vi "layout.vi"(0 "reference":refnum<class "PackageNode.lvclass">, 1 "graph":refnum<class "Graph.lvclass">, 2 "graphics":refnum<class "Graphics.lvclass">, 3 "grid":refnum<class "Grid.lvclass">, 5 "error in (no error)":errorcluster) -> (14 "reference out":refnum<class "PackageNode.lvclass">, 19 "error out":errorcluster)   [LabVIEW 2020, in "PackageNode.lvclass"]
doc: "public void draw(Graphics2D g2)"
uses:
  <resource>/Framework/Providers/Open_GDS/UML/PackageNode_class/PackageNode.lvclass
  C:/Program Files (x86)/National Instruments/LabVIEW 2020/resource/Framework/Providers/Open_GDS/UML/RectangularNode_class/RectangularNode.lvclass
  C:/Program Files (x86)/National Instruments/LabVIEW 2020/resource/Framework/Providers/Open_GDS/UML/AbstractNode_class/AbstractNode.lvclass
  <resource>/Framework/Providers/Open_GDS/UML/Grid_class/Grid.lvclass
  <resource>/Framework/Providers/Open_GDS/UML/Graphics_class/Graphics.lvclass
  <resource>/Framework/Providers/Open_GDS/UML/Graph_class/Graph.lvclass
  <resource>/Framework/Providers/Open_GDS/UML/General/Rectangle/Rectangle Rectangle2D.ctl
  <resource>/Framework/Providers/Open_GDS/UML/MultiLineString_class/MultiLineString.lvclass
  <resource>/Framework/Providers/Open_GDS/UML/AbstractNode_class/AbstractNode.lvclass
  <resource>/Framework/Providers/Open_GDS/UML/RectangularNode_class/RectangularNode.lvclass
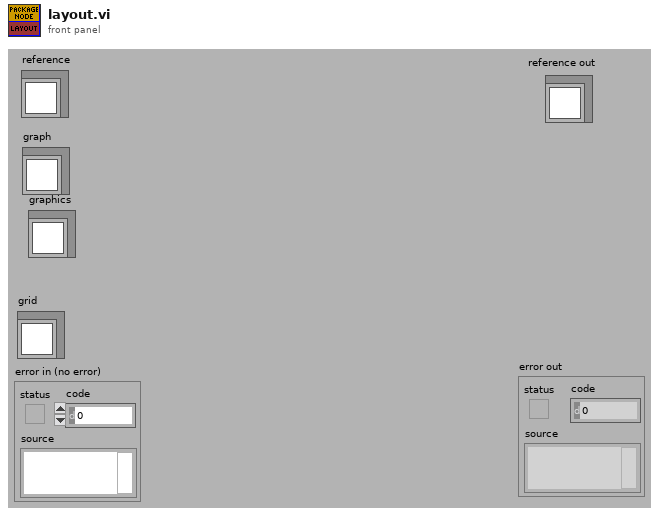
[diagram p1: front panel]
types:
  T1 = typedef "Rectangle Rectangle2D.ctl" = cluster{"x":dbl, "y":dbl, "width":dbl, "height":dbl}
  T2 = typedef "PackageNode.lvclass/ObjectAttributes.ctl" = cluster{"name":string, "contents":refnum<class "MultiLineString.lvclass">, "DEFAULT_TOP_WIDTH":i32, "DEFAULT_TOP_HEIGHT":i32, "DEFAULT_WIDTH":i32, "DEFAULT_HEIGHT":i32, "NAME_GAP":i32, "XGAP":i32, "YGAP":i32, "Collapsed":bool, "Note color":u32, "Justification":u16}
  T3 = typedef "RectangularNode.lvclass/ObjectAttributes.ctl" = cluster{"bounds":T1}
  T4 = typedef "AbstractNode.lvclass/ObjectAttributes.ctl" = cluster{"parent":refnum<class "AbstractNode.lvclass">, "children":refnum<class "AbstractNode.lvclass">[], "Hidden":bool}
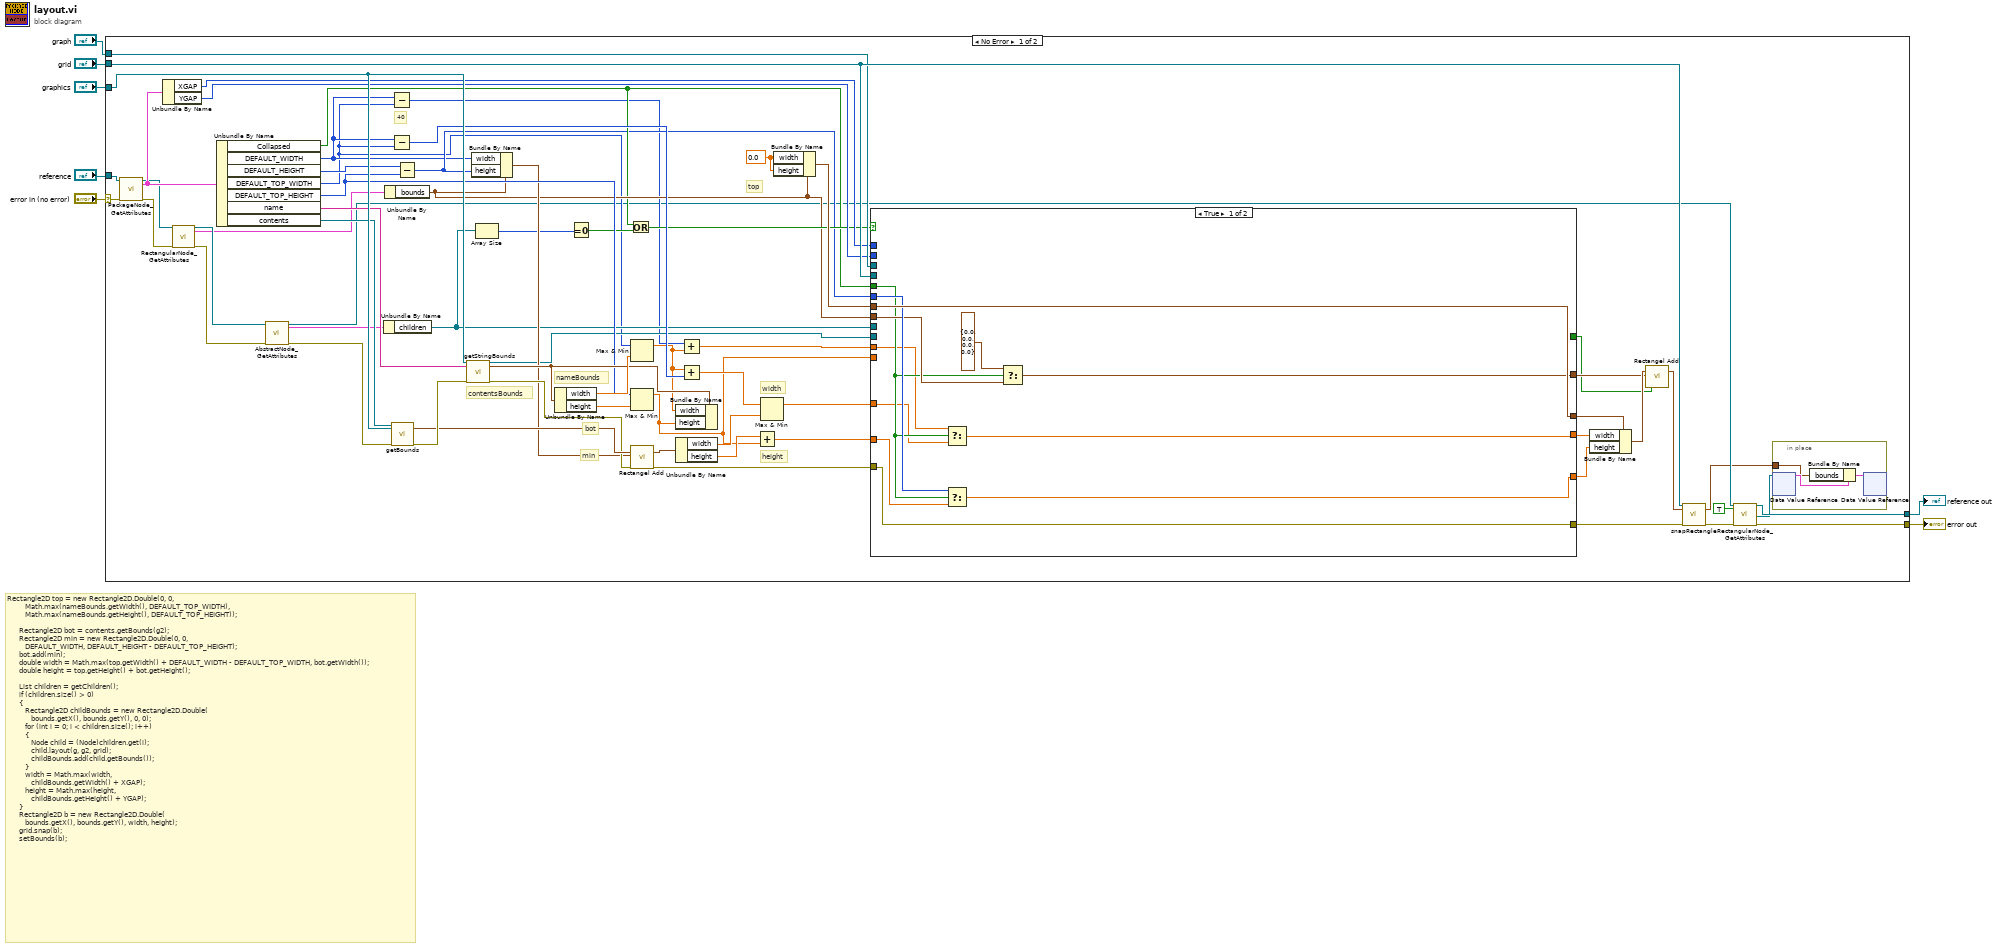
[diagram p0: block diagram]
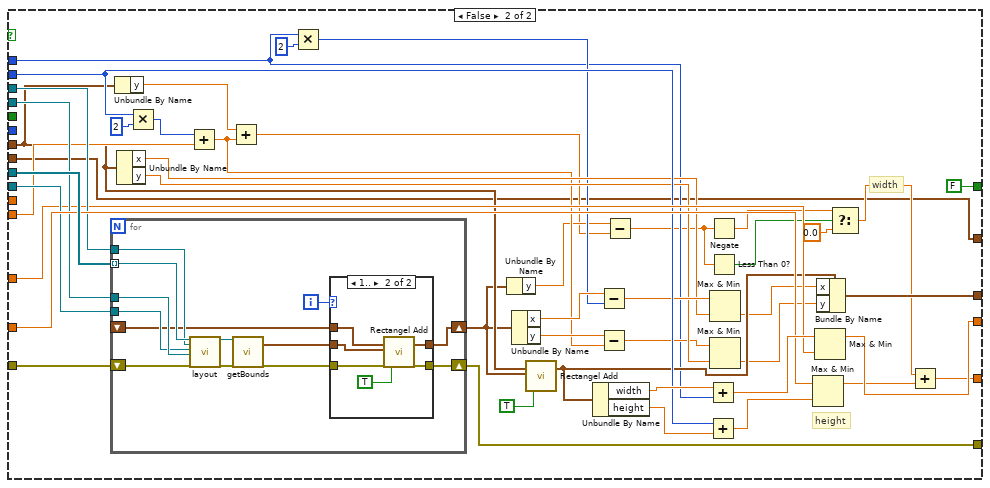
[diagram p2: hidden frame]
diagram:
  # "Rectangle2D top = new Rectangle2D.Double(0, 0,\n         Math.max(nameBounds.getWidth(), DEFAULT_TOP_WIDTH), \n         Math.max(nameBounds.getHeight(), DEFAULT_TOP_HEIGHT));\n\n      Rectangle2D bot = contents.getBounds(g2);\n      Rectangle2D min = new Rectangle2D.Double(0, 0,\n         DEFAULT_WIDTH, DEFAULT_HEIGHT - DEFAULT_TOP_HEIGHT);\n      bot.add(min);\n      double width = Math.max(top.getWidth() + DEFAULT_WIDTH - DEFAULT_TOP_WIDTH, bot.getWidth());\n      double height = top.getHeight() + bot.getHeight();\n\n      List children = getChildren();\n      if (children.size() > 0)\n      {\n         Rectangle2D childBounds = new Rectangle2D.Double(\n            bounds.getX(), bounds.getY(), 0, 0);\n         for (int i = 0; i < children.size(); i++)\n         {\n            Node child = (Node)children.get(i);\n            child.layout(g, g2, grid);\n            childBounds.add(child.getBounds());\n         }\n         width = Math.max(width, \n            childBounds.getWidth() + XGAP);\n         height = Math.max(height, \n            childBounds.getHeight() + YGAP);\n      }\n      Rectangle2D b = new Rectangle2D.Double(\n         bounds.getX(), bounds.getY(), width, height);\n      grid.snap(b);\n      setBounds(b);"
  n1 = case shown="No Error" "error in (no error)" {
    selector: "error in (no error)" -> [w35 w155]
    tunnel: "reference" -> [w72 w156]
    tunnel: [w71 w155] -> w6
    tunnel: [w70 w156] -> w5
    tunnel: "graphics" -> [w69 _]
    tunnel: "grid" -> [w68 _]
    tunnel: "graph" -> [w67 _]
    frame No Error {
      w45 = 0.0 ("width")
      # "40"
      # "height"
      # "width"
      # "bot"
      # "min"
      # "contentsBounds"
      # "top"
      # "nameBounds"
      n2 = call <resource>:"PackageNode_GetAttributes.vi"("reference in"=w72, "error in (no error)"=w35) -> ("reference out"=w17:refnum<class "PackageNode.lvclass">, "Data"=w18:T2, "error out"=w16:errorcluster)  [unwired: 1 in, 14 out]
      n3 = Unbundle By Name(w18) -> ("XGAP"=w44:i32, "YGAP"=w43:i32)
      n4 = call <resource>:"RectangularNode_GetAttributes.vi"("reference in"=w17, "error in (no error)"=w16) -> ("reference out"=w15:refnum<class "PackageNode.lvclass">, "Data"=w10:T3, "error out"=w14:errorcluster)  [unwired: 14 in, 1 out]
      n5 = Unbundle By Name(w18) -> ("Collapsed"=w27:bool, "DEFAULT_WIDTH"=w24:i32, "DEFAULT_HEIGHT"=w58:i32, "DEFAULT_TOP_WIDTH"=w23:i32, "DEFAULT_TOP_HEIGHT"=w57:i32, "name"=w62:string, "contents"=w64:refnum<class "MultiLineString.lvclass">)
      n6 = call <resource>:"AbstractNode_GetAttributes.vi"("reference in"=w15, "error in (no error)"=w14) -> ("reference out"=w12:refnum<class "PackageNode.lvclass">, "Data"=w11:T4, "error out"=w13:errorcluster)  [unwired: 14 in, 1 out]
      n7 = Unbundle By Name(w11) -> ("children"=w49:refnum<class "AbstractNode.lvclass">[])
      n8 = Unbundle By Name(w10) -> ("bounds"=w29:T1)
      n9 = Subtract(x=w24, y=w23) -> (x-y=w21:i32)
      n10 = Subtract(x=w24, y=w23) -> (x-y=w52:i32)
      n11 = call-dynamic "getBounds.vi"("reference"=w64, "graphics"=w69, "error in (no error)"=w13) -> ("bounds"=w61:T1, "error out"=w63:errorcluster)  [unwired: 14 in, 1 out]
      n12 = Subtract(x=w58, y=w57) -> (x-y=w26:i32)
      n13 = call-dynamic "getStringBounds.vi"("reference"=w69, "text"=w62, "error in (no error)"=w63) -> ("reference out"=w39:refnum<class "Graphics.lvclass">, "bounds"=w59:T1, "error out"=w60:errorcluster)  [unwired: 14 in]
      n14 = Bundle By Name(cluster=w29, "width"=w24, "height"=w26) -> (w56:T1)
      n15 = Array Size(array=w49) -> (size(s)=w32:i32)
      n16 = Unbundle By Name(w59) -> ("width"=w66:dbl, "height"=w65:dbl)
      n17 = Equal To 0?(x=w32) -> (x = 0?=w31:bool)
      n18 = Or(x=w27, y=w31) -> (x .or. y?=w30:bool)
      n19 = Max & Min(x=w23, y=w66) -> (max(x,y)=w22:dbl)  [unwired: 1 out]
      n20 = Max & Min(x=w57, y=w65) -> (max(x,y)=w36:dbl)  [unwired: 1 out]
      n21 = call <resource>:"Rectangel Add.vi"("bounds1"=w61, "bounds2"=w56, "error in (no error)"=w60) -> ("boundsAdded"=w55:T1, "error out"=w50:errorcluster)  [unwired: 2 in, 13 out]
      n22 = Bundle By Name(cluster=w59, "width"=w22, "height"=w36) -> ()  [unwired: 1 out]
      n23 = Unbundle By Name(w55) -> ("width"=w54:dbl, "height"=w51:dbl)
      n24 = Add(x=w21, y=w22) -> (x+y=w20:dbl)
      n25 = Add(x=w22, y=w52) -> (x+y=w53:dbl)
      n26 = Add(x=w51, y=w36) -> (x+y=w47:dbl)
      n27 = Max & Min(x=w53, y=w54) -> (max(x,y)=w48:dbl)  [unwired: 1 out]
      n28 = Bundle By Name(cluster=w29, "width"=w45, "height"=w45) -> (w37:T1)
      n29 = case shown="True" w30 {
        tunnel: w50 -> [w87 w133]
        tunnel: w49 -> [_ w132]
        tunnel: w48 -> [w78 w120]
        tunnel: w47 -> [w85 w129]
        tunnel: w37 -> [w86 w102]
        tunnel: w44 -> [_ w103]
        tunnel: w43 -> [_ w119]
        tunnel: [w77 w126] -> w42
        tunnel: [w84 w96] -> w41
        tunnel: [w87 w125] -> w40
        tunnel: w68 -> [_ w124]
        tunnel: w39 -> [_ w123]
        tunnel: w67 -> [_ w122]
        tunnel: [w86 w113] -> w38
        tunnel: w36 -> [_ w116]
        tunnel: w29 -> [w81 w89]
        tunnel: [w82 w89] -> w28
        tunnel: w27 -> [w79 _]
        tunnel: w26 -> [w83 _]
        tunnel: [_ FALSE ("useAbsoluteCordinates(False)")] -> w25
        tunnel: w20 -> [w76 _]
        frame True {
          n30 = Select(t=w76, s=w79, f=w78) -> (s? t:f=w77:dbl)
          n31 = Select(t=w83, s=w79, f=w85) -> (s? t:f=w84:dbl)
          n32 = Select(t=T1 {"x"=0.0, "y"=0.0, "width"=0.0, "height"=0.0}, s=w79, f=w81) -> (s? t:f=w82:T1)
        }
        frame False {
          # "height"
          # "width"
          n33 = for {
            tunnel: w132 -> [w144] mode=indexing
            shift-right: [w146] -> w125
            shift-left: w133 -> [w145]
            shift-right: [w140] -> w101
            shift-left: _ -> [w136]
            tunnel: w124 -> [w139]
            tunnel: w123 -> [w138]
            tunnel: w122 -> [w137]
            i -> [w134]
            n34 = call-dynamic "layout.vi"("reference"=w144, "graph"=w137, "graphics"=w138, "grid"=w139, "error in (no error)"=w145) -> ("reference out"=w143:refnum<class "AbstractNode.lvclass">, "error out"=w142:errorcluster)  [unwired: 13 in]
            n35 = call-dynamic "getBounds.vi"("reference"=w143, "error in (no error)"=w142) -> ("bounds"=w135:T1, "error out"=w141:errorcluster)  [unwired: 15 in, 1 out]
            n36 = case shown="1.." w134 {
              tunnel: [w148 w154] -> w146
              tunnel: w141 -> [w148 w153]
              tunnel: [w147 w152] -> w140
              tunnel: w136 -> [_ w151]
              tunnel: w135 -> [w147 w150]
              frame 0, Default {
              }
              frame 1.. {
                n37 = call <resource>:"Rectangel Add.vi"("bounds1"=w151, "bounds2"=w150, "error in (no error)"=w153, "useAbsoluteCordinates(False)"=TRUE) -> ("boundsAdded"=w152:T1, "error out"=w154:errorcluster)  [unwired: 1 in, 13 out]
              }
            }
          }
          n38 = Unbundle By Name(w102) -> ("y"=w100:dbl)
          n39 = Unbundle By Name(w102) -> ("x"=w109:dbl, "y"=w108:dbl)
          n40 = Multiply(x=w119, y=2) -> (x*y=w117:i32)
          n41 = Add(x=w117, y=w116) -> (x+y=w99:dbl)
          n42 = Add(x=w100, y=w99) -> (x+y=w97:dbl)
          n43 = Multiply(x=w103, y=2) -> (x*y=w104:i32)
          n44 = Unbundle By Name(w101) -> ("y"=w98:dbl)
          n45 = Unbundle By Name(w101) -> ("x"=w115:dbl, "y"=w121:dbl)
          n46 = call <resource>:"Rectangel Add.vi"("bounds1"=w102, "bounds2"=w101, "useAbsoluteCordinates(False)"=TRUE) -> ("boundsAdded"=w112:T1)  [unwired: 2 in, 14 out]
          n47 = Unbundle By Name(w112) -> ("width"=w131:dbl, "height"=w128:dbl)
          n48 = Subtract(x=w115, y=w104) -> (x-y=w111:dbl)
          n49 = Subtract(x=w121, y=w99) -> (x-y=w107:dbl)
          n50 = Subtract(x=w98, y=w97) -> (x-y=w92:dbl)
          n51 = Add(x=w131, y=w103) -> (x+y=w130:dbl)
          n52 = Add(x=w119, y=w128) -> (x+y=w127:dbl)
          n53 = Negate(x=w92) -> (-x=w91:dbl)
          n54 = Less Than 0?(x=w92) -> (x < 0?=w94:bool)
          n55 = Max & Min(x=w111, y=w109) -> (min(x,y)=w110:dbl)  [unwired: 1 out]
          n56 = Max & Min(x=w107, y=w108) -> (min(x,y)=w106:dbl)  [unwired: 1 out]
          n57 = Max & Min(x=w129, y=w127) -> (max(x,y)=w95:dbl)  [unwired: 1 out]
          n58 = Max & Min(x=w130, y=w120) -> (max(x,y)=w126:dbl)  [unwired: 1 out]
          n59 = Bundle By Name(cluster=w112, "x"=w110, "y"=w106) -> (w113:T1)
          n60 = Select(t=w91, s=w94, f=0.0) -> (s? t:f=w93:dbl)
          n61 = Add(x=w93, y=w95) -> (x+y=w96:dbl)
        }
      }
      n62 = Bundle By Name(cluster=w38, "width"=w42, "height"=w41) -> (w34:T1)
      n63 = call <resource>:"Rectangel Add.vi"("bounds1"=w34, "bounds2"=w28, "useAbsoluteCordinates(False)"=w25) -> ("boundsAdded"=w33:T1)  [unwired: 2 in, 14 out]
      n64 = call <resource>:"snapRectangle.vi"("reference"=w68, "bounds"=w33, "error in (no error)"=w40) -> ("boundsOut"=w8:T1, "error out"=w46:errorcluster)  [unwired: 15 out]
      n65 = call <resource>:"RectangularNode_GetAttributes.vi"("reference in"=w12, "OnlyGetDvrReference(False)"=TRUE, "error in (no error)"=w46) -> ("reference out"=w70:refnum<class "PackageNode.lvclass">, "DataRef"=w9:refnum<data-value>, "error out"=w71:errorcluster)  [unwired: 13 in, 1 out]
      n66 = in-place {
        in-place-border: w8 -> [w74]
        n67 = in-place-dvr #1(w9) -> (w75:T3)  [unwired: 1 out]
        n68 = Bundle By Name(cluster=w75, "bounds"=w74) -> (w73:T3)
        n69 = in-place-dvr #1(w73) -> ()  [unwired: 2 out]
      }
    }
    frame Error {
    }
  }
  "reference out" <- w5
  "error out" <- w6
